vi "GetParameterInfo.vi"(7 "Camera Parameter":T2, 8 "error in (no error)":errorcluster, 11 "Stream in":refnum<class "Stream.lvclass">) -> (0 "error out":errorcluster, 2 "Info":T1, 3 "Stream (Duplicate)":refnum<class "Stream.lvclass">)   [LabVIEW 2020, in "g_ar_toolkit.capture.lvlib" / "Stream.lvclass"]
uses:
  Stream.lvclass
  Camera Parameters.ctl
  Camera Parameter Information.ctl
  Stream.lvclass/Stream.ctl
  g_ar_toolkit.common/g_ar_toolkit.common.lvlib
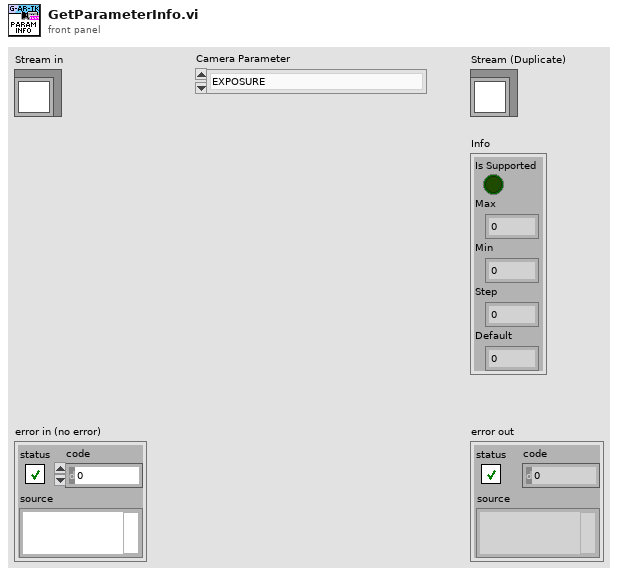
[diagram p1: front panel]
types:
  T1 = typedef "g_ar_toolkit.capture.lvlib/Stream.lvclass/Camera Parameter Information.ctl" = cluster{"Is Supported":bool, "Max":i32, "Min":i32, "Step":i32, "Default":i32}
  T2 = typedef "g_ar_toolkit.capture.lvlib/Stream.lvclass/Camera Parameters.ctl" = enum8{"EXPOSURE", "FOCUS", "ZOOM", "GAIN", "WHITE_BALANCE_TEMPERATURE", "BRIGHTNESS", "CONTRAST", "SATURATION", "GAMMA", "HUE", "SHARPNESS", "BACKLIGHT_COMPENSATION", "POWER_LINE_FREQUENCY"}
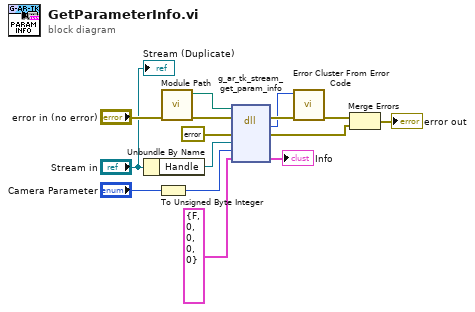
[diagram p0: block diagram]
diagram:
  n1 = Unbundle By Name("Stream in") -> ("Handle"=w12:refnum<data-value>)
  n2 = To Unsigned Byte Integer(number="Camera Parameter") -> (unsigned 8bit integer=w5:u8)
  n3 = call "Module Path.vi"("error in (no error)"="error in (no error)") -> ("error out"=w2:errorcluster, "Path"=w1:path)  [unwired: 9 in]
  n4 = dll-call lib="?" fn="g_ar_tk_stream_get_param_info" ("g_ar_toolkit.*.*:g_ar_tk_stream_capture_next")(path in=w1, error in=w2, "error_cluster"=errorcluster {"status"=FALSE, "code"=0, "source"=""} ("error constant"), "EDVR_strm"=w12, "parameter"=w5, "info"=T1 {"Is Supported"=FALSE, "Max"=0, "Min"=0, "Step"=0, "Default"=0} ("Camera Parameter Information")) -> (error out=w11:errorcluster, "MgErr"=w10:i32, "error_cluster"=w8:errorcluster, "info"=→"Info":T1)  [unwired: 3 in, 1 out]
  n5 = call <vilib>:"Error Cluster From Error Code.vi"("error in (no error)"=w11, "error code (0)"=w10) -> ("error out"=w9:errorcluster)  [unwired: 7 in]
  n6 = Merge Errors(w9, w8) -> (→"error out":errorcluster)
  "Stream (Duplicate)" <- "Stream in"
